vi "WriteDataVariant.vi"(8 "error in (no error)":errorcluster, 10 "DataVariant":variant, 11 "Singleton.lvclass In":refnum<class "Singleton.lvclass">) -> (0 "error out":errorcluster, 3 "SingletonDVR Out":refnum<data-value>)   [LabVIEW 2013, in "Singleton.lvclass"]
uses:
  Singleton.lvclass
  Singleton.lvclass/Singleton.ctl
panel:
  # "WriteDataVariant"
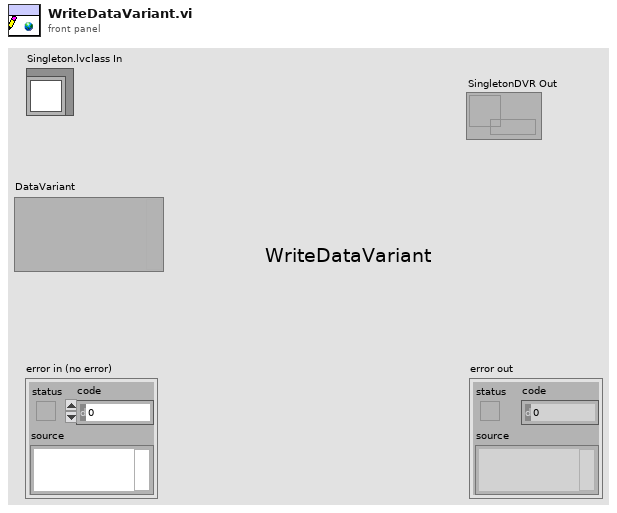
[diagram p1: front panel]
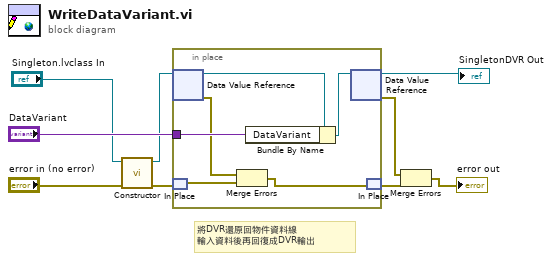
[diagram p0: block diagram]
diagram:
  # "將DVR還原回物件資料線\n輸入資料後再回復成DVR輸出"
  n1 = call "Constructor.vi"("error in (no error)"="error in (no error)", "Singleton.lvclass In"="Singleton.lvclass In") -> ("error out"=w3:errorcluster, "SingletonDVR Out"=w2:refnum<data-value>)  [unwired: 8 in]
  n2 = in-place {
    in-place-border: "DataVariant" -> [w15]
    n3 = in-place-dvr #1(w2) -> (w14:refnum<class "Singleton.lvclass">, w11:errorcluster)
    n4 = in-place-match #2(w3) -> (w12:errorcluster)
    n5 = Merge Errors(w11, w12) -> (w10:errorcluster)
    n6 = Bundle By Name(cluster=w14, "DataVariant"=w15) -> (w13:refnum<class "Singleton.lvclass">)
    n7 = in-place-dvr #1(w13) -> (→"SingletonDVR Out":refnum<data-value>, w6:errorcluster)
    n8 = in-place-match #2(w10) -> (w7:errorcluster)
  }
  n9 = Merge Errors(w6, w7) -> (→"error out":errorcluster)
